vi "ValChange.vi"(6 "Value":string, 8 "error in (no error)":errorcluster, 9 "Table CtlRef In":refnum<vi>, 10 "Cell Position":T1, 11 "Column in":refnum<class "Column.lvclass">) -> (0 "error out":errorcluster, 1 "Table CtlRef Out":refnum<vi>, 3 "Column out":refnum<class "Column.lvclass">)   [LabVIEW 2013, in "Column.lvclass"]
doc: "If a table cell value changes, calling this method will ensure the change is pushed down to any subsequent disabled cells.\nThis is read only w.r.t. column data (only for dynamic dispatch)."
uses:
  Column.lvclass
  <vilib>/Utility/miscctls.llb/LVRowAndColumnTypeDef.ctl
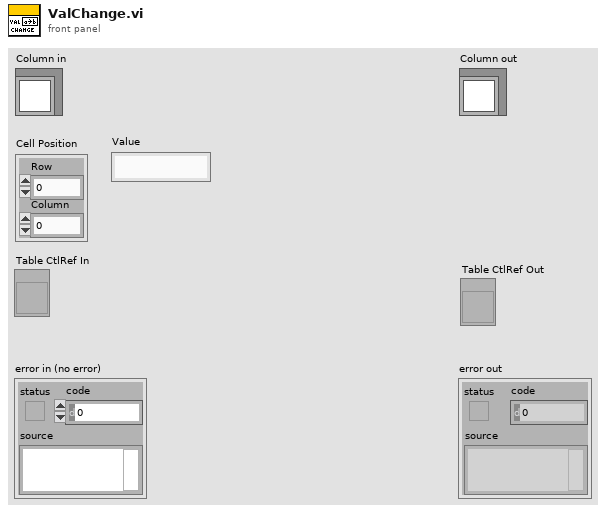
[diagram p1: front panel]
types:
  T1 = typedef "LVRowAndColumnTypeDef.ctl" = cluster{"Row":i32, "Column":i32}
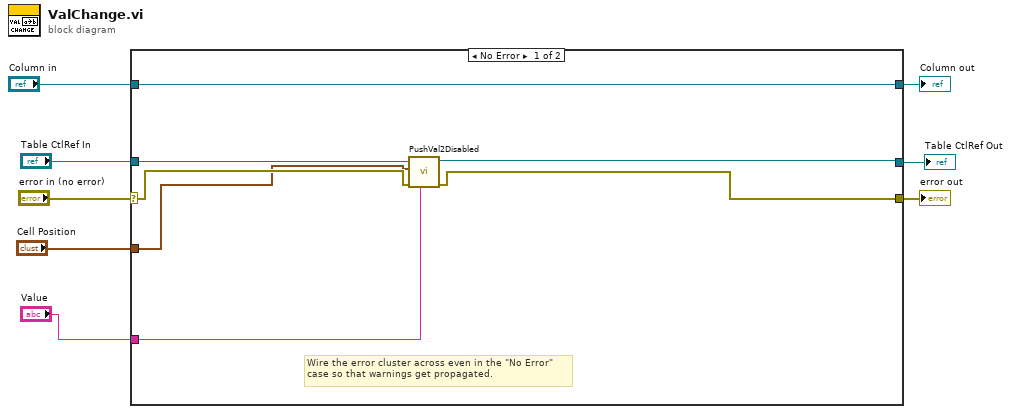
[diagram p0: block diagram]
diagram:
  n1 = case shown="No Error" "error in (no error)" {
    selector: "error in (no error)" -> [w13 w18]
    tunnel: [w9 w18] -> w7
    tunnel: [w15 w17] -> w5
    tunnel: "Column in" -> [w15 w17]
    tunnel: [w10 w16] -> w4
    tunnel: "Table CtlRef In" -> [w14 w16]
    tunnel: "Cell Position" -> [w12 _]
    tunnel: "Value" -> [w11 _]
    frame No Error {
      # "Wire the error cluster across even in the \"No Error\"\ncase so that warnings get propagated."
      n2 = call "PushVal2Disabled.vi"("Value"=w11, "error in (no error)"=w13, "Cell Position"=w12, "Table CtlRef In"=w14) -> ("error out"=w9:errorcluster, "Table CtlRef Out"=w10:refnum<vi>)  [unwired: 5 in, 1 out]
    }
    frame Error {
    }
  }
  "error out" <- w7
  "Column out" <- w5
  "Table CtlRef Out" <- w4
